vi "Init.vi"(10 "Attributes":T1) -> (3 "Base Attributes out":refnum<class "Base Attributes.lvclass">)   [LabVIEW 2025, in "jettl.lvlib" / "Attributes.lvlib" / "Base Attributes.lvclass"]
uses:
  Base Attributes.lvclass
  Base Attributes.lvclass/Base Attributes.ctl
  Msg/Msg.lvclass
  Msg Set.ctl
  jettl.lvlib
  Attributes.ctl
  Transport/Transport/Transport.lvclass
  Attributes/Attributes.lvclass
  Actor/Actor.lvclass
  Refs/Refs.lvclass
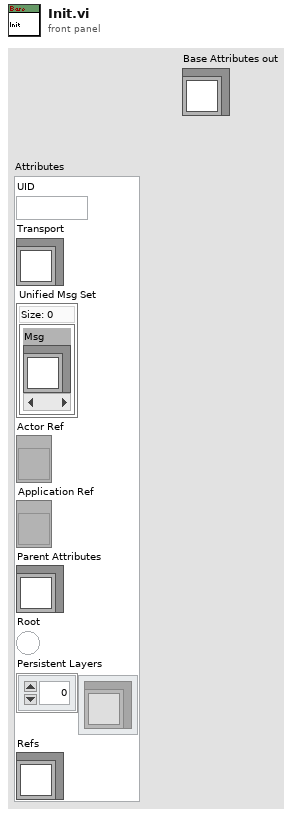
[diagram p1: front panel]
types:
  T1 = typedef "jettl.lvlib/Attributes.ctl" = cluster{"UID":string, "Transport":refnum<class "Transport.lvclass">, "Unified Msg Set":T2, "Actor Ref":refnum<vi>, "Application Ref":refnum<vi>, "Parent Attributes":refnum<class "Attributes.lvclass">, "Root":bool, "Persistent Layers":refnum<class "Actor.lvclass">[], "Refs":refnum<class "Refs.lvclass">}
  T2 = typedef "jettl.lvlib/Msg Set.ctl" = set{refnum<class "Msg.lvclass">}
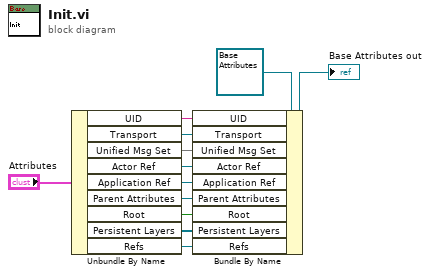
[diagram p0: block diagram]
diagram:
  n1 = Unbundle By Name("Attributes") -> ("UID"=w5:string, "Transport"=w6:refnum<class "Transport.lvclass">, "Unified Msg Set"=w7:T2, "Actor Ref"=w8:refnum<vi>, "Application Ref"=w9:refnum<vi>, "Parent Attributes"=w4:refnum<class "Attributes.lvclass">, "Root"=w3:bool, "Persistent Layers"=w2:refnum<class "Actor.lvclass">[], "Refs"=w1:refnum<class "Refs.lvclass">)
  n2 = Bundle By Name(cluster=refnum<class "Base Attributes.lvclass"> refnum ("Base Attributes in"), "UID"=w5, "Transport"=w6, "Unified Msg Set"=w7, "Actor Ref"=w8, "Application Ref"=w9, "Parent Attributes"=w4, "Root"=w3, "Persistent Layers"=w2, "Refs"=w1) -> (→"Base Attributes out":refnum<class "Base Attributes.lvclass">)
